vi "PositionUpDown.vi"   [LabVIEW 2016, in "Gear Manipulator.lvclass"]
uses:
  Gear Manipulator.lvclass
  Gear Manipulator.lvclass/Gear Manipulator.ctl
  <vilib>/Rock Robotics/WPI/Solenoid/WPI_SolenoidValue.ctl
  GearManipulatorSingleton.vi
  <vilib>/Rock Robotics/WPI/Solenoid/WPI_SolenoidSetEnum.vi
types:
  T1 = typedef "WPI_SolenoidValue.ctl" = enum16{"Off", "On", "Forward", "Reverse"}
  T2 = typedef "WPI_SolenoidDevRef.ctl" = cluster{"DevStatus":errorcluster, "Pneumatics Control Module":u8, "Forward Solenoid Channel":T3, "Reverse Solenoid Channel":T3}
  T3 = typedef "WPI_SolenoidChannel.ctl" = enum8{"Solenoid 0", "Solenoid 1", "Solenoid 2", "Solenoid 3", "Solenoid 4", "Solenoid 5", "Solenoid 6", "Solenoid 7", "Invalid"}
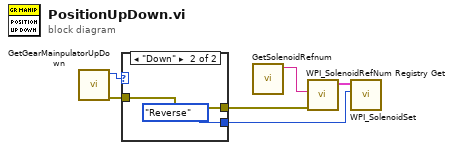
[diagram p0: block diagram]
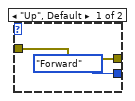
[diagram p2: hidden frame]
diagram:
  n1 = call "GetGearMainpulatorUpDown.vi"() -> ("error out"=w2:errorcluster, "Gear Mainpulator Up Down"=w3:enum16{"Up", "Down"})  [unwired: 10 in]
  n2 = case shown="\"Down\"" w3 {
    tunnel: [WPI_SolenoidValue."Forward" ("Value") WPI_SolenoidValue."Reverse" ("Value")] -> w6
    tunnel: [w7 w9] -> w1
    tunnel: w2 -> [w7 w9]
    frame "Up", Default {
    }
    frame "Down" {
    }
  }
  n3 = call "GetSolenoidRefnum.vi"() -> ("OpenCloseSolenoidRefnum"=w5:string)  [unwired: 10 in, 1 out]
  n4 = call <vilib>:"WPI_SolenoidRefNum Registry Get.vi"("error in (no error)"=w1, "refnum name"=w5) -> ("SolenoidDevRef"=w4:T2)  [unwired: 8 in, 1 out]
  n5 = call-poly <vilib>:"WPI_SolenoidSet.vi"("Value"=w6, "SolenoidDevRef"=w4) -> ()  [unwired: 8 in, 2 out]
